vi "Remove First and Last.vi"(1 "Char to Remove":string, 2 "String":string) -> (0 "Result":string)   [LabVIEW 2019, in "Useful HTTP VIs.lvlib"]
uses:
  Useful HTTP VIs/Useful HTTP VIs.lvlib
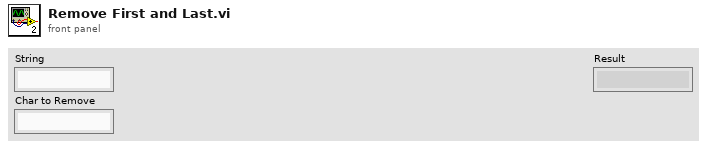
[diagram p1: front panel]
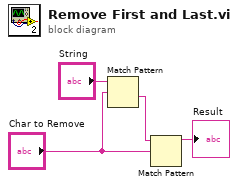
[diagram p0: block diagram]
diagram:
  n1 = Match Pattern(string="String", regular expression="Char to Remove") -> (after substring=w3:string)  [unwired: 1 in, 3 out]
  n2 = Match Pattern(string=w3, regular expression="Char to Remove") -> (before substring=→"Result":string)  [unwired: 1 in, 3 out]
